vi "MPU_Stick_UI_Indicators_Updator.vi"(8 "error in (no error)":errorcluster, 11 "MPU_Stick_Globals":T1) -> ()   [LabVIEW 2017]
uses:
  Controls/MPU_Stick_Globals.ctl
  Controls/IMU_Configuration_References.ctl
  Controls/MP_Comp_Filter_Constants_References.ctl
  Controls/MD_Threshold_References.ctl
  Controls/MD_Type_References.ctl
  Controls/LED_Configuration_References.ctl
  Controls/Primary_References.ctl
  Controls/MPU_Stick_Queues.ctl
  Controls/MPU_Stick_Queue_Element.ctl
  Controls/MPU_Stick_Queue_Commands.ctl
  Classes/ADCP.lvclass
  Controls/MPU_Stick_Timestamped_Data.ctl
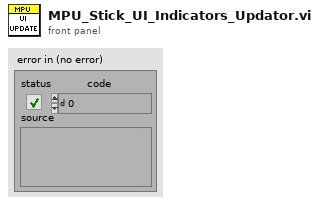
[diagram p1: front panel]
types:
  T1 = typedef "MPU_Stick_Globals.ctl" = cluster{"IMU_configuration_references":T2, "MP_Comp_Filter_Constants_References":T3, "MD_Threshold_References":T4, "MD_Type_References":T5, "LED_Configuration_References":T6, "Primary_references":T7, "MPU_Stick_Queues":T8, "ADCP":refnum<vi>}
  T2 = typedef "IMU_Configuration_References.ctl" = cluster{"Get all IMU configurations":refnum<vi>, "Set all IMU configurations":refnum<vi>, "Get sampling frequency":refnum<vi>, "Set sampling frequency":refnum<vi>, "Get calibration point count":refnum<vi>, "Set calibration point count":refnum<vi>, "Get calibration interval":refnum<vi>, "Set calibration interval":refnum<vi>, "Get Gyroscope bandwidth":refnum<vi>, "Set Gyroscope bandwidth":refnum<vi>, "Get Gyroscope F.S. Value":refnum<vi>, "Set Gyroscope F.S. Value":refnum<vi>, "Get Accelerometer bandwidth":refnum<vi>, "Set Accelerometer bandwidth":refnum<vi>, "Get Accelerometer F.S. Value":refnum<vi>, "Set Accelerometer F.S. Value":refnum<vi>, "Sampling frequency (Hz)":refnum<vi>, "Calibration point count":refnum<vi>, "Calibration interval (ms)":refnum<vi>, "IMU Gyroscope bandwidth":refnum<vi>, "IMU Gyroscope F.S. value":refnum<vi>, "IMU Accelerometer bandwidth":refnum<vi>, "IMU Accelerometer F.S. value":refnum<vi>}
  T3 = typedef "MP_Comp_Filter_Constants_References.ctl" = cluster{"Set pitch filter constant":refnum<vi>, "Get pitch filter constant":refnum<vi>, "Set roll filter constant":refnum<vi>, "Get roll filter constant":refnum<vi>, "Pitch filter constant":refnum<vi>, "Roll filter constant":refnum<vi>}
  T4 = typedef "MD_Threshold_References.ctl" = cluster{"Yaw threshold (U)":refnum<vi>, "Yaw threshold (L)":refnum<vi>, "Pitch threshold (U)":refnum<vi>, "Pitch. threshold (L)":refnum<vi>, "Roll threshold (U)":refnum<vi>, "Roll threshold (L)":refnum<vi>, "Z gyro. threshold (U)":refnum<vi>, "Z gyro. threshold (L)":refnum<vi>, "Y gyro. threshold (U)":refnum<vi>, "Y gyro. threshold (L)":refnum<vi>, "X gyro. threshold (U)":refnum<vi>, "X gyro. threshold (L)":refnum<vi>, "Z accel. threshold (U)":refnum<vi>, "Z accel. threshold (L)":refnum<vi>, "Y accel. threshold (U)":refnum<vi>, "Y accel. threshold (L)":refnum<vi>, "X accel. threshold (U)":refnum<vi>, "X accel. threshold (L)":refnum<vi>, "Set all Motion detection threshold configurations":refnum<vi>, "Get yaw threshold (upper)":refnum<vi>, "Get yaw threshold (lower)":refnum<vi>, "Get pitch threshold (upper)":refnum<vi>, "Get pitch threshold (lower)":refnum<vi>, "Get roll threshold (upper)":refnum<vi>, "Get roll threshold (lower)":refnum<vi>, "Get Z gyro threshold (upper)":refnum<vi>, "Get Z gyro threshold (lower)":refnum<vi>, "Get Y gyro threshold (upper)":refnum<vi>, "Get Y gyro threshold (lower)":refnum<vi>, "Get X gyro threshold (upper)":refnum<vi>, "Get X gyro threshold (lower)":refnum<vi>, "Get Z accel threshold (upper)":refnum<vi>, "Get Z accel threshold (lower)":refnum<vi>, "Get Y accel threshold (upper)":refnum<vi>, "Get Y accel threshold (lower)":refnum<vi>, "Get X accel threshold (upper)":refnum<vi>, "Get X accel threshold (lower)":refnum<vi>, "Get all Motion detection threshold configurations":refnum<vi>, "Set yaw threshold (upper)":refnum<vi>, "Set yaw threshold (lower)":refnum<vi>, "Set pitch threshold (upper)":refnum<vi>, "Set pitch threshold (lower)":refnum<vi>, "Set roll threshold (upper)":refnum<vi>, "Set roll threshold (lower)":refnum<vi>, "Set Z gyro threshold (upper)":refnum<vi>, "Set Z gyro threshold (lower)":refnum<vi>, "Set Y gyro threshold (upper)":refnum<vi>, "Set Y gyro threshold (lower)":refnum<vi>, "Set X gyro threshold (upper)":refnum<vi>, "Set X gyro threshold (lower)":refnum<vi>, "Set Z accel threshold (upper)":refnum<vi>, "Set Z accel threshold (lower)":refnum<vi>, "Set Y accel threshold (upper)":refnum<vi>, "Set Y accel threshold (lower)":refnum<vi>, "Set X accel threshold (upper)":refnum<vi>, "Set X accel threshold (lower)":refnum<vi>}
  T5 = typedef "MD_Type_References.ctl" = cluster{"Yaw threshold type":refnum<vi>, "Pitch threshold type":refnum<vi>, "Roll threshold type":refnum<vi>, "Z gyro threshold type":refnum<vi>, "Y gyro threshold type":refnum<vi>, "X gyro threshold type":refnum<vi>, "Z accel threshold type":refnum<vi>, "Y accel threshold type":refnum<vi>, "X accel threshold type":refnum<vi>, "Set all Motion detection type configurations":refnum<vi>, "Get all Motion detection type configurations":refnum<vi>, "Set yaw threshold type":refnum<vi>, "Get yaw threshold type":refnum<vi>, "Set pitch threshold type":refnum<vi>, "Get pitch threshold type":refnum<vi>, "Set roll threshold type":refnum<vi>, "Get roll threshold type":refnum<vi>, "Set Z gyroscope threshold type":refnum<vi>, "Get Z gyroscope threshold type":refnum<vi>, "Set Y gyroscope threshold type":refnum<vi>, "Get Y gyroscope threshold type":refnum<vi>, "Set X gyroscope threshold type":refnum<vi>, "Get X gyroscope threshold type":refnum<vi>, "Set Z accel threshold type":refnum<vi>, "Get Z accel threshold type":refnum<vi>, "Set Y accel threshold type":refnum<vi>, "Get Y accel threshold type":refnum<vi>, "Get X accel threshold type":refnum<vi>, "Set X accel threshold type":refnum<vi>}
  T6 = typedef "LED_Configuration_References.ctl" = cluster{"Get all LED configurations":refnum<vi>, "Set all LED configurations":refnum<vi>, "Get LED3 configuration":refnum<vi>, "Set LED3 configuration":refnum<vi>, "Get LED2 configuration":refnum<vi>, "Set LED2 configuration":refnum<vi>, "Get LED1 configuration":refnum<vi>, "Set LED1 configuration":refnum<vi>, "LED3 Configuration":refnum<vi>, "LED2 Configuration":refnum<vi>, "LED1 Configuration":refnum<vi>}
  T7 = typedef "Primary_References.ctl" = cluster{"3D View Image":refnum<vi>, "Plot":refnum<vi>, "Graph / 3D view tab control":refnum<vi>, "MP Reset":refnum<vi>, "Calibrate IMU":refnum<vi>, "Plot Parameter List":refnum<vi>, "Remove Parameter from Plot":refnum<vi>, "Add Parameter to Plot":refnum<vi>, "Parameter to monitor":refnum<vi>, "Yaw motion detection output":refnum<vi>, "Pitch motion detection output":refnum<vi>, "Roll motion detection output":refnum<vi>, "Z gyro motion detection output":refnum<vi>, "Y gyro motion detection output":refnum<vi>, "X gyro motion detection output":refnum<vi>, "Z accel motion detection output":refnum<vi>, "Y accel motion detection output":refnum<vi>, "X accel motion detection output":refnum<vi>, "Yaw angle (filter) (degrees)":refnum<vi>, "Pitch angle (filter) (degrees)":refnum<vi>, "Roll angle (filter) (degrees)":refnum<vi>, "Yaw angle (gyro) (degrees)":refnum<vi>, "Pitch angle (gyro) (degrees)":refnum<vi>, "Roll angle (gyro) (degrees)":refnum<vi>, "Yaw angle (accel) (degrees)":refnum<vi>, "Pitch angle (accel) (degrees)":refnum<vi>, "Roll angle (accel) (degrees)":refnum<vi>, "Z gyroscope reading (DPS)":refnum<vi>, "Y gyroscope reading (DPS)":refnum<vi>, "X gyroscope reading (DPS)":refnum<vi>, "Z accelerometer reading (G)":refnum<vi>, "Y accelerometer reading (G)":refnum<vi>, "X accelerometer reading (G)":refnum<vi>, "Save all config.":refnum<vi>, "Write all config.":refnum<vi>, "Read all config.":refnum<vi>, "Tab Control":refnum<vi>, "Baud Rate":refnum<vi>, "COM Port":refnum<vi>, "Time (ms)":refnum<vi>, "Value (Units)":refnum<vi>, "Exit Application":refnum<vi>, "Connect Device":refnum<vi>, "Progress Bar":refnum<vi>, "Get Range & Offset":refnum<vi>, "Range":refnum<vi>, "Offset":refnum<vi>, "Set Range & Offset":refnum<vi>, "Parameter name":refnum<vi>, "Plot time (ms)":refnum<vi>, "Plot value":refnum<vi>}
  T8 = typedef "MPU_Stick_Queues.ctl" = cluster{"UI Event Handler":refnum<queue>, "3D View Updater":refnum<queue>, "Plot Updater":refnum<queue>, "Serial Port Reader":refnum<queue>, "UI Indicators Updater":refnum<queue>}
  T9 = typedef "MPU_Stick_Timestamped_Data.ctl" = cluster{"Parameter name":string, "Time (ms)":dbl, "Value":dbl}
  T10 = typedef "MPU_Stick_Queue_Element.ctl" = cluster{"Data":variant, "Command":T11}
  T11 = typedef "MPU_Stick_Queue_Commands.ctl" = enum16{"UI_Event_Exit_Application_RQST", "UI_Event_Exit_Application_ACK", "UI_Event_Connect_Device_RQST", "UI_Event_Connect_Device_ACK", "UI_Event_Disconnect_Device_RQST", "UI_Event_Disconnect_Device_ACK", "UI_Event_Read_All_Configurations_RQST", "UI_Event_Read_All_Configurations_ACK", "UI_Event_Write_All_Configurations_RQST", "UI_Event_Write_All_Configurations_ACK", "UI_Event_Save_All_Configurations_RQST", "UI_Event_Save_All_Configurations_ACK", "UI_Event_Calibrate_IMU_Sensor_RQST", "UI_Event_Calibrate_IMU_Sensor_ACK", "UI_Event_MP_Reset_RQST", "UI_Event_MP_Reset_ACK", "UI_Event_Get_Config_RQST", "UI_Event_Get_Config_ACK", "UI_Event_Set_Config_RQST", "UI_Event_Set_Config_ACK", "Read_Serial_Port_Data_Pause", "Read_Serial_Port_Data_Pause_ACK", "Read_Serial_Port_Data_Continue", "Read_Serial_Port_Data_Exit", "Plotter_Exit", "Plotter_Update", "Plotter_Add_Channel", "Plotter_Remove_Channel", "3D Viewer Update", "3D Viewer Exit", "UI Indicators Update", "UI Indicators Exit"}
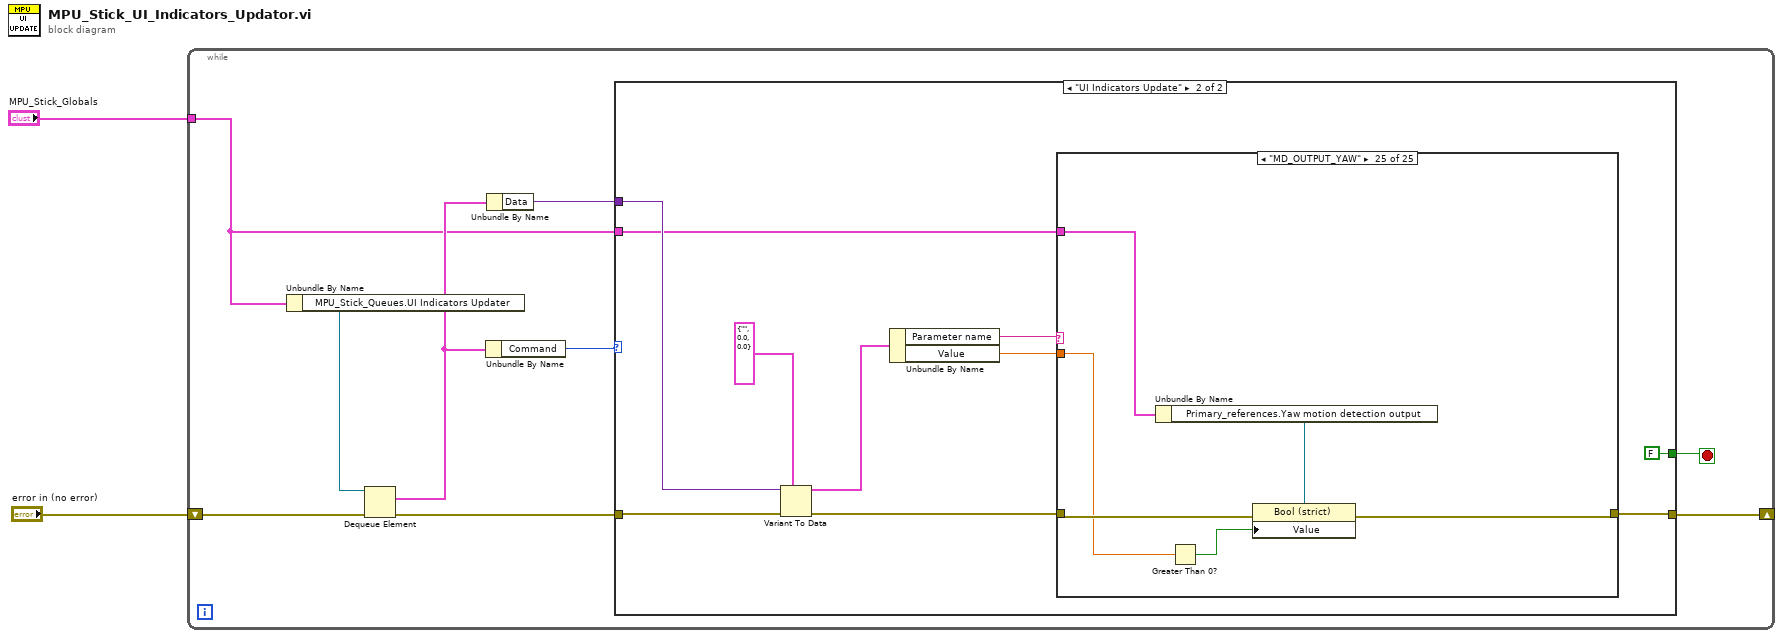
[diagram p0: block diagram]
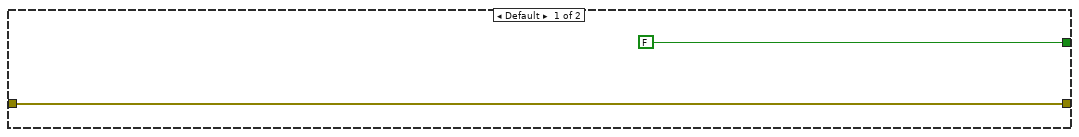
[diagram p2: hidden frame]
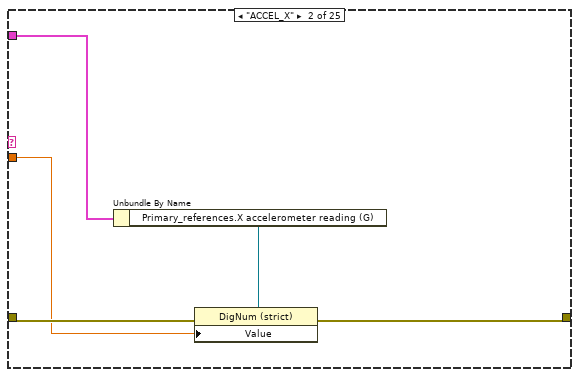
[diagram p4: hidden frame]
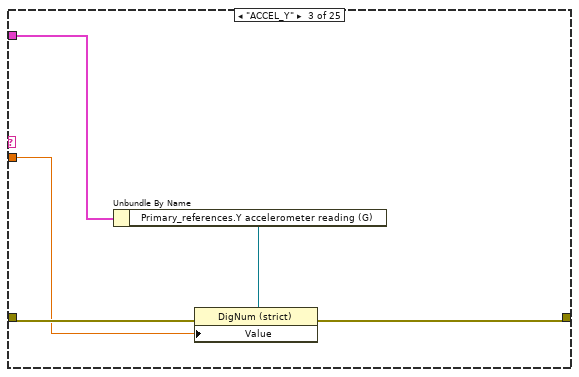
[diagram p5: hidden frame]
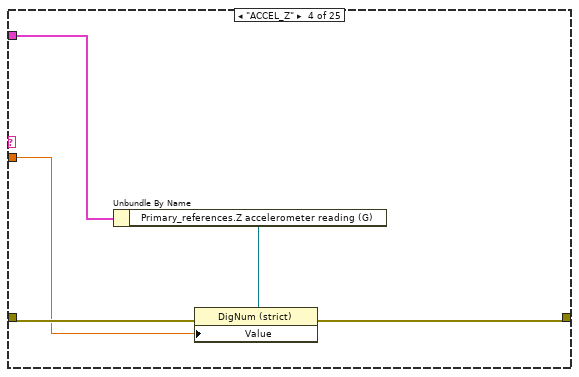
[diagram p6: hidden frame]
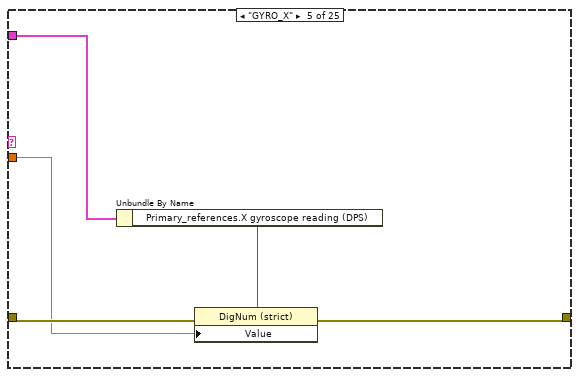
[diagram p7: hidden frame]
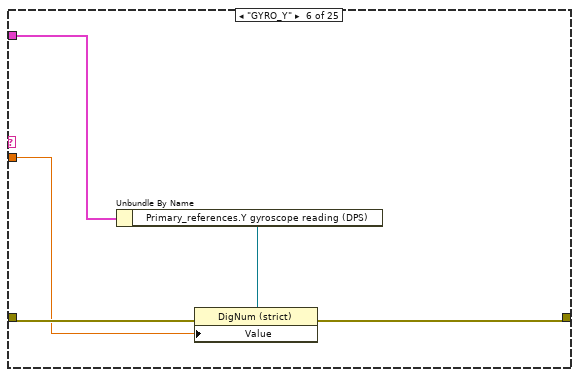
[diagram p8: hidden frame]
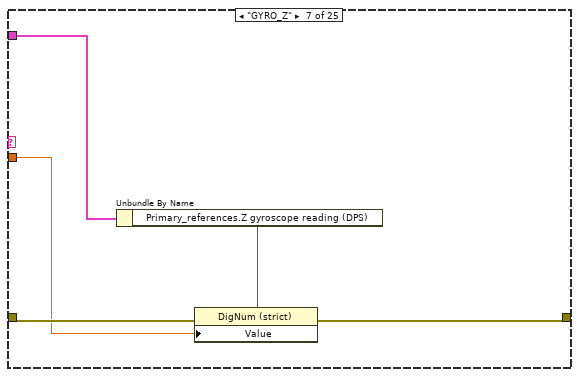
[diagram p9: hidden frame]
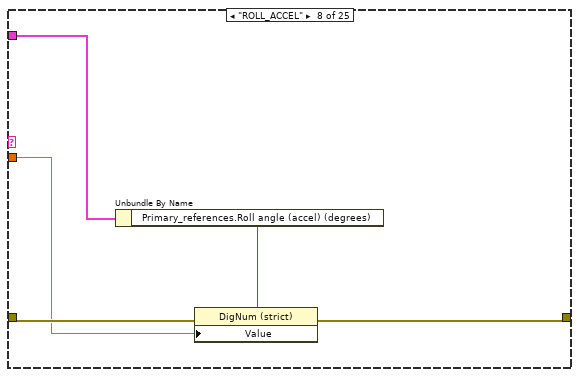
[diagram p10: hidden frame]
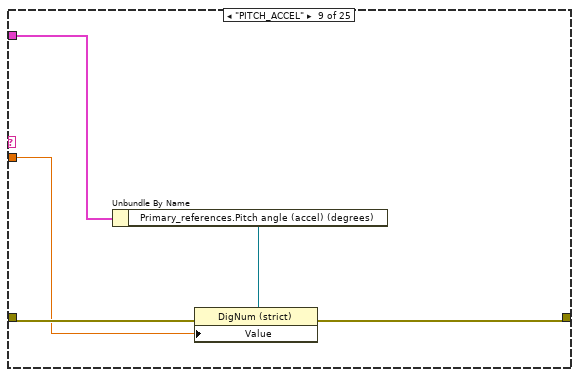
[diagram p11: hidden frame]
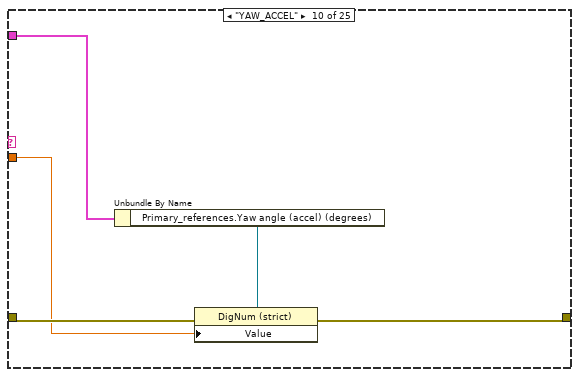
[diagram p12: hidden frame]
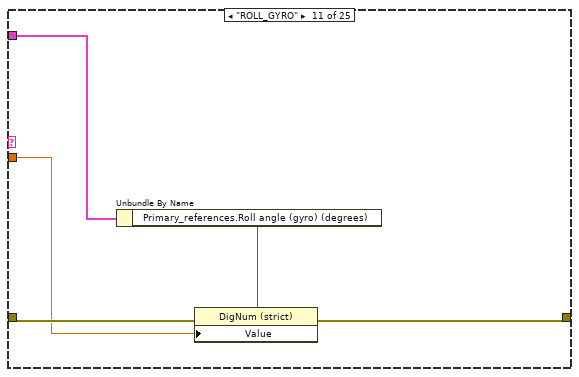
[diagram p13: hidden frame]
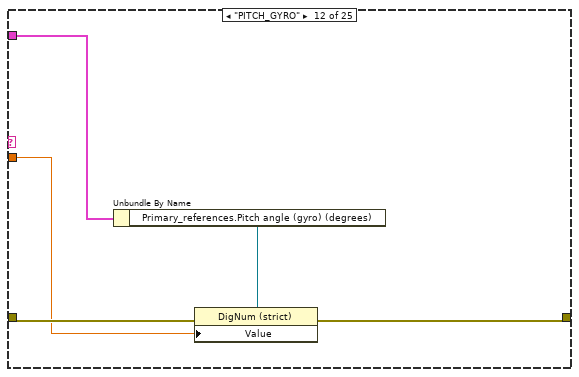
[diagram p14: hidden frame]
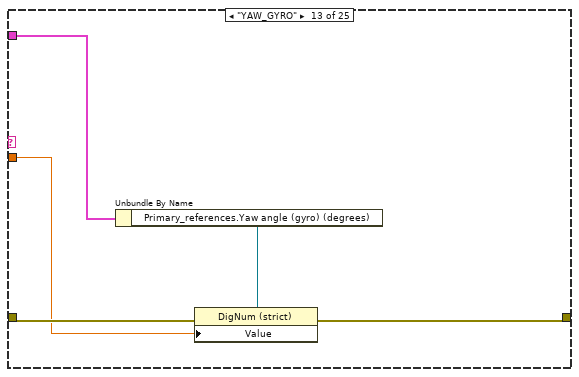
[diagram p15: hidden frame]
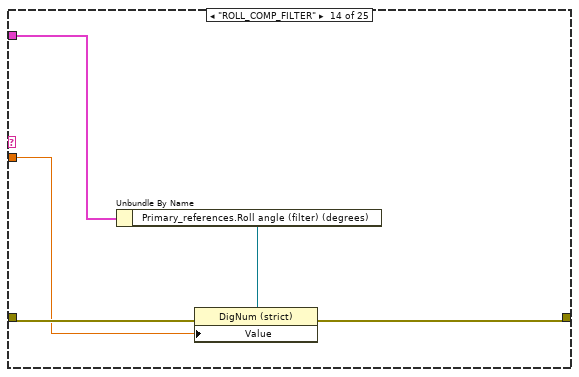
[diagram p16: hidden frame]
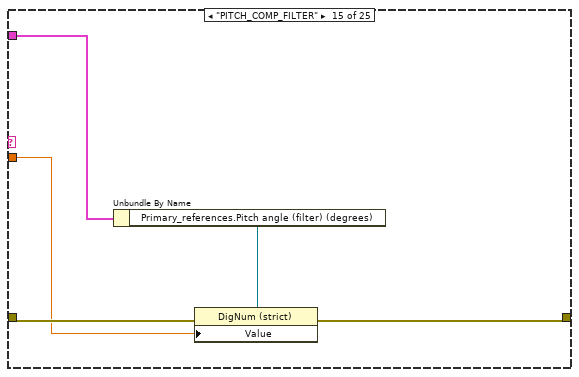
[diagram p17: hidden frame]
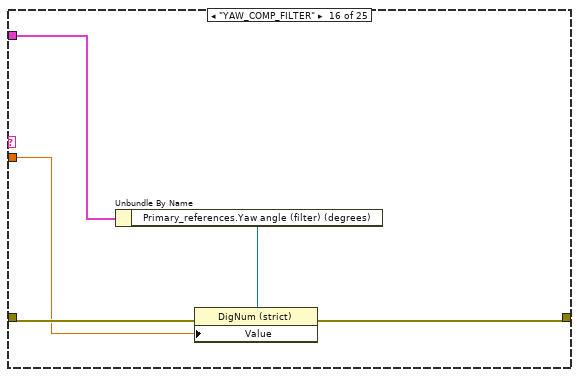
[diagram p18: hidden frame]
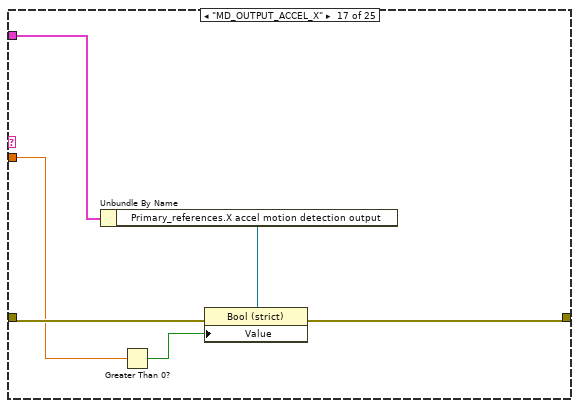
[diagram p19: hidden frame]
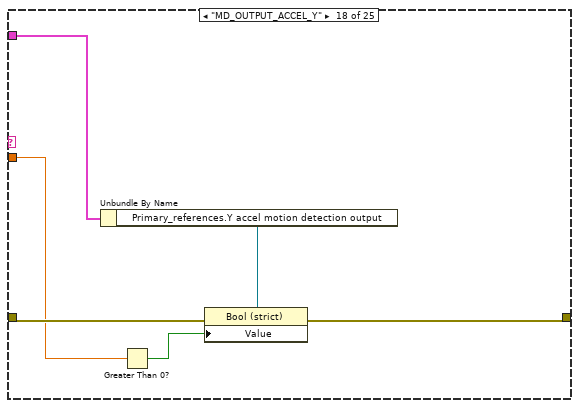
[diagram p20: hidden frame]
diagram:
  n1 = while {
    tunnel: "MPU_Stick_Globals" -> [w3]
    shift-right: [w6] -> _
    shift-left: "error in (no error)" -> [w11]
    stop <- w7 stop-if-true
    n2 = Unbundle By Name(w3) -> ("MPU_Stick_Queues.UI Indicators Updater"=w10:refnum<queue>)
    n3 = Dequeue Element(queue=w10, error in (no error)=w11) -> (element=w5:T10, error out=w9:errorcluster)  [unwired: 1 in, 2 out]
    n4 = Unbundle By Name(w5) -> ("Command"=w8:T11)
    n5 = Unbundle By Name(w5) -> ("Data"=w4:variant)
    n6 = case shown="\"UI Indicators Update\"" w8 {
      tunnel: w9 -> [w12 w22]
      tunnel: [FALSE FALSE] -> w7
      tunnel: [w12 w15] -> w6
      tunnel: w4 -> [_ w21]
      tunnel: w3 -> [_ w14]
      frame Default {
      }
      frame "UI Indicators Update" {
        n7 = Variant To Data(error in=w22, type=T9 {"Parameter name"="", "Time (ms)"=0.0, "Value"=0.0} ("Cluster"), Variant=w21) -> (data=w19:T9, error out=w16:errorcluster)
        n8 = Unbundle By Name(w19) -> ("Parameter name"=w18:string, "Value"=w17:dbl)
        n9 = case shown="\"MD_OUTPUT_YAW\"" w18 {
          tunnel: w17 -> [_ w25 w30 w35 w40 w45 w50 w55 w60 w65 w70 w75 w80 w85 w90 w95 w101 w107 w113 w119 w125 w131 w137 w143 w149]
          tunnel: w16 -> [w24 w27 w32 w37 w42 w47 w52 w57 w62 w67 w72 w77 w82 w87 w92 w97 w103 w109 w115 w121 w127 w133 w139 w145 w151]
          tunnel: [w24 w26 w31 w36 w41 w46 w51 w56 w61 w66 w71 w76 w81 w86 w91 w96 w102 w108 w114 w120 w126 w132 w138 w144 w150] -> w15
          tunnel: w14 -> [_ w29 w34 w39 w44 w49 w54 w59 w64 w69 w74 w79 w84 w89 w94 w99 w105 w111 w117 w123 w129 w135 w141 w147 w153]
          frame Default {
          }
          frame "ACCEL_X" {
            n10 = Unbundle By Name(w29) -> ("Primary_references.X accelerometer reading (G)"=w28:refnum<vi>)
            n11 = property class="DigNum (strict)"(reference=w28, error in=w27, "Value"=w25) -> (error out=w26:errorcluster)  [unwired: 1 out]
          }
          frame "ACCEL_Y" {
            n12 = Unbundle By Name(w34) -> ("Primary_references.Y accelerometer reading (G)"=w33:refnum<vi>)
            n13 = property class="DigNum (strict)"(reference=w33, error in=w32, "Value"=w30) -> (error out=w31:errorcluster)  [unwired: 1 out]
          }
          frame "ACCEL_Z" {
            n14 = Unbundle By Name(w39) -> ("Primary_references.Z accelerometer reading (G)"=w38:refnum<vi>)
            n15 = property class="DigNum (strict)"(reference=w38, error in=w37, "Value"=w35) -> (error out=w36:errorcluster)  [unwired: 1 out]
          }
          frame "GYRO_X" {
            n16 = Unbundle By Name(w44) -> ("Primary_references.X gyroscope reading (DPS)"=w43:refnum<vi>)
            n17 = property class="DigNum (strict)"(reference=w43, error in=w42, "Value"=w40) -> (error out=w41:errorcluster)  [unwired: 1 out]
          }
          frame "GYRO_Y" {
            n18 = Unbundle By Name(w49) -> ("Primary_references.Y gyroscope reading (DPS)"=w48:refnum<vi>)
            n19 = property class="DigNum (strict)"(reference=w48, error in=w47, "Value"=w45) -> (error out=w46:errorcluster)  [unwired: 1 out]
          }
          frame "GYRO_Z" {
            n20 = Unbundle By Name(w54) -> ("Primary_references.Z gyroscope reading (DPS)"=w53:refnum<vi>)
            n21 = property class="DigNum (strict)"(reference=w53, error in=w52, "Value"=w50) -> (error out=w51:errorcluster)  [unwired: 1 out]
          }
          frame "ROLL_ACCEL" {
            n22 = Unbundle By Name(w59) -> ("Primary_references.Roll angle (accel) (degrees)"=w58:refnum<vi>)
            n23 = property class="DigNum (strict)"(reference=w58, error in=w57, "Value"=w55) -> (error out=w56:errorcluster)  [unwired: 1 out]
          }
          frame "PITCH_ACCEL" {
            n24 = Unbundle By Name(w64) -> ("Primary_references.Pitch angle (accel) (degrees)"=w63:refnum<vi>)
            n25 = property class="DigNum (strict)"(reference=w63, error in=w62, "Value"=w60) -> (error out=w61:errorcluster)  [unwired: 1 out]
          }
          frame "YAW_ACCEL" {
            n26 = Unbundle By Name(w69) -> ("Primary_references.Yaw angle (accel) (degrees)"=w68:refnum<vi>)
            n27 = property class="DigNum (strict)"(reference=w68, error in=w67, "Value"=w65) -> (error out=w66:errorcluster)  [unwired: 1 out]
          }
          frame "ROLL_GYRO" {
            n28 = Unbundle By Name(w74) -> ("Primary_references.Roll angle (gyro) (degrees)"=w73:refnum<vi>)
            n29 = property class="DigNum (strict)"(reference=w73, error in=w72, "Value"=w70) -> (error out=w71:errorcluster)  [unwired: 1 out]
          }
          frame "PITCH_GYRO" {
            n30 = Unbundle By Name(w79) -> ("Primary_references.Pitch angle (gyro) (degrees)"=w78:refnum<vi>)
            n31 = property class="DigNum (strict)"(reference=w78, error in=w77, "Value"=w75) -> (error out=w76:errorcluster)  [unwired: 1 out]
          }
          frame "YAW_GYRO" {
            n32 = Unbundle By Name(w84) -> ("Primary_references.Yaw angle (gyro) (degrees)"=w83:refnum<vi>)
            n33 = property class="DigNum (strict)"(reference=w83, error in=w82, "Value"=w80) -> (error out=w81:errorcluster)  [unwired: 1 out]
          }
          frame "ROLL_COMP_FILTER" {
            n34 = Unbundle By Name(w89) -> ("Primary_references.Roll angle (filter) (degrees)"=w88:refnum<vi>)
            n35 = property class="DigNum (strict)"(reference=w88, error in=w87, "Value"=w85) -> (error out=w86:errorcluster)  [unwired: 1 out]
          }
          frame "PITCH_COMP_FILTER" {
            n36 = Unbundle By Name(w94) -> ("Primary_references.Pitch angle (filter) (degrees)"=w93:refnum<vi>)
            n37 = property class="DigNum (strict)"(reference=w93, error in=w92, "Value"=w90) -> (error out=w91:errorcluster)  [unwired: 1 out]
          }
          frame "YAW_COMP_FILTER" {
            n38 = Unbundle By Name(w99) -> ("Primary_references.Yaw angle (filter) (degrees)"=w98:refnum<vi>)
            n39 = property class="DigNum (strict)"(reference=w98, error in=w97, "Value"=w95) -> (error out=w96:errorcluster)  [unwired: 1 out]
          }
          frame "MD_OUTPUT_ACCEL_X" {
            n40 = Unbundle By Name(w105) -> ("Primary_references.X accel motion detection output"=w104:refnum<vi>)
            n41 = Greater Than 0?(x=w101) -> (x > 0?=w100:bool)
            n42 = property class="Bool (strict)"(reference=w104, error in=w103, "Value"=w100) -> (error out=w102:errorcluster)  [unwired: 1 out]
          }
          frame "MD_OUTPUT_ACCEL_Y" {
            n43 = Unbundle By Name(w111) -> ("Primary_references.Y accel motion detection output"=w110:refnum<vi>)
            n44 = Greater Than 0?(x=w107) -> (x > 0?=w106:bool)
            n45 = property class="Bool (strict)"(reference=w110, error in=w109, "Value"=w106) -> (error out=w108:errorcluster)  [unwired: 1 out]
          }
          frame "MD_OUTPUT_ACCEL_Z" {
            n46 = Unbundle By Name(w117) -> ("Primary_references.Z accel motion detection output"=w116:refnum<vi>)
            n47 = Greater Than 0?(x=w113) -> (x > 0?=w112:bool)
            n48 = property class="Bool (strict)"(reference=w116, error in=w115, "Value"=w112) -> (error out=w114:errorcluster)  [unwired: 1 out]
          }
          frame "MD_OUTPUT_GYRO_X" {
            n49 = Unbundle By Name(w123) -> ("Primary_references.X gyro motion detection output"=w122:refnum<vi>)
            n50 = Greater Than 0?(x=w119) -> (x > 0?=w118:bool)
            n51 = property class="Bool (strict)"(reference=w122, error in=w121, "Value"=w118) -> (error out=w120:errorcluster)  [unwired: 1 out]
          }
          frame "MD_OUTPUT_GYRO_Y" {
            n52 = Unbundle By Name(w129) -> ("Primary_references.Y gyro motion detection output"=w128:refnum<vi>)
            n53 = Greater Than 0?(x=w125) -> (x > 0?=w124:bool)
            n54 = property class="Bool (strict)"(reference=w128, error in=w127, "Value"=w124) -> (error out=w126:errorcluster)  [unwired: 1 out]
          }
          frame "MD_OUTPUT_GYRO_Z" {
            n55 = Unbundle By Name(w135) -> ("Primary_references.Z gyro motion detection output"=w134:refnum<vi>)
            n56 = Greater Than 0?(x=w131) -> (x > 0?=w130:bool)
            n57 = property class="Bool (strict)"(reference=w134, error in=w133, "Value"=w130) -> (error out=w132:errorcluster)  [unwired: 1 out]
          }
          frame "MD_OUTPUT_ROLL" {
            n58 = Unbundle By Name(w141) -> ("Primary_references.Roll motion detection output"=w140:refnum<vi>)
            n59 = Greater Than 0?(x=w137) -> (x > 0?=w136:bool)
            n60 = property class="Bool (strict)"(reference=w140, error in=w139, "Value"=w136) -> (error out=w138:errorcluster)  [unwired: 1 out]
          }
          frame "MD_OUTPUT_PITCH" {
            n61 = Unbundle By Name(w147) -> ("Primary_references.Pitch motion detection output"=w146:refnum<vi>)
            n62 = Greater Than 0?(x=w143) -> (x > 0?=w142:bool)
            n63 = property class="Bool (strict)"(reference=w146, error in=w145, "Value"=w142) -> (error out=w144:errorcluster)  [unwired: 1 out]
          }
          frame "MD_OUTPUT_YAW" {
            n64 = Unbundle By Name(w153) -> ("Primary_references.Yaw motion detection output"=w152:refnum<vi>)
            n65 = Greater Than 0?(x=w149) -> (x > 0?=w148:bool)
            n66 = property class="Bool (strict)"(reference=w152, error in=w151, "Value"=w148) -> (error out=w150:errorcluster)  [unwired: 1 out]
          }
        }
      }
    }
  }
